vi "Exit.vi"(7 "Main VI":refnum<vi>, 8 "Error In":errorcluster, 9 "Messages":refnum<queue>, 10 "User Event In":refnum<user-event>, 11 "State In":T1) -> (0 "Error Out":errorcluster, 2 "User Event Out":refnum<user-event>, 3 "State Out":T1)   [LabVIEW 2018, in "Bookmark Manager.lvlib"]
uses:
  Bookmark Manager.lvlib
  Controls/State.ctl
  <vilib>/addons/analyzer/_analyzerctrls.llb/VIAnCtl Analysis App Info.ctl
  Controls/Bookmark.ctl
  Controls/VI Identifier.ctl
  Controls/Bookmarks Groups.ctl
  Controls/Message.ctl
  <vilib>/event_ctls.llb/usereventprio.ctl
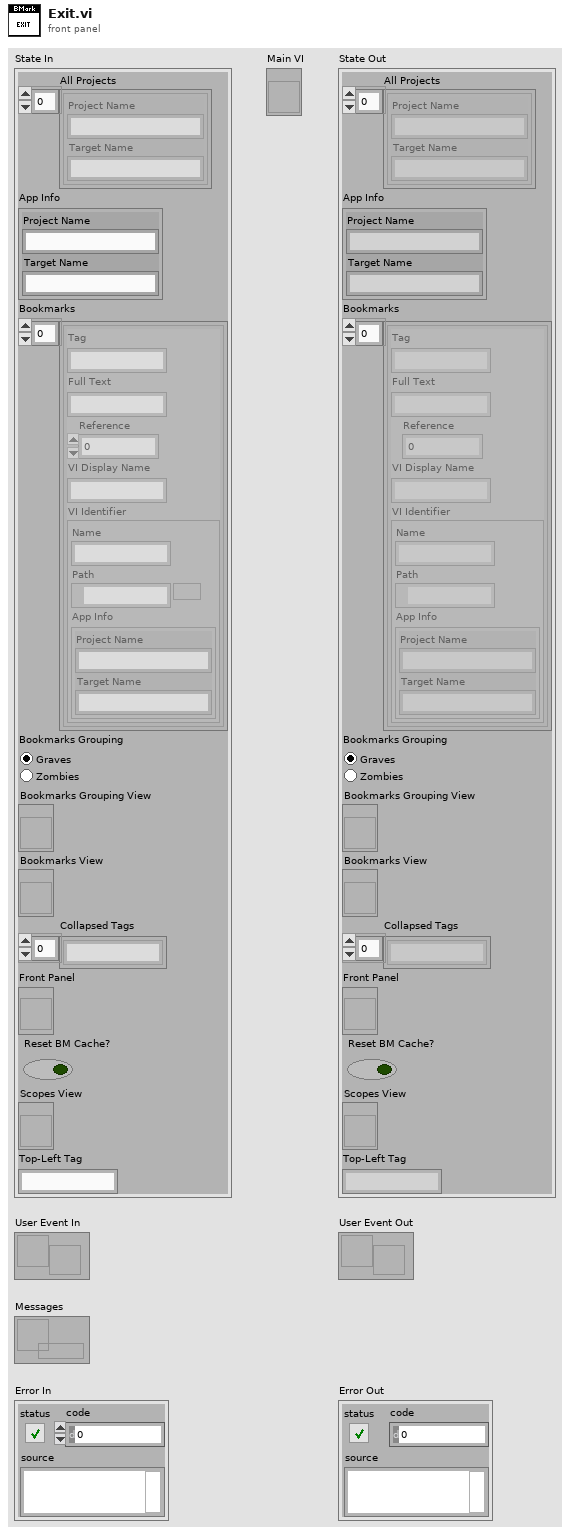
[diagram p1: front panel]
types:
  T1 = typedef "Bookmark Manager.lvlib/State.ctl" = cluster{"All Projects":T2[], "App Info":T2, "Bookmarks":T3[], "Bookmarks Grouping":T5, "Bookmarks Grouping View":refnum<vi>, "Bookmarks View":refnum<vi>, "Collapsed Tags":string[], "Front Panel":refnum<vi>, "Reset BM Cache?":bool, "Scopes View":refnum<vi>, "Top-Left Tag":string}
  T2 = typedef "VIAnCtl Analysis App Info.ctl" = cluster{"Project Name":string, "Target Name":string}
  T3 = typedef "Bookmark Manager.lvlib/Bookmark.ctl" = cluster{"Tag":string, "Full Text":string, "Reference":i32, "VI Display Name":string, "VI Identifier":T4}
  T4 = typedef "Bookmark Manager.lvlib/VI Identifier.ctl" = cluster{"Name":string, "Path":path, "App Info":T2}
  T5 = typedef "Bookmark Manager.lvlib/Bookmarks Groups.ctl" = enum32{"Graves", "Zombies"}
  T6 = typedef "usereventprio.ctl" = enum32{"high priority", "normal priority"}
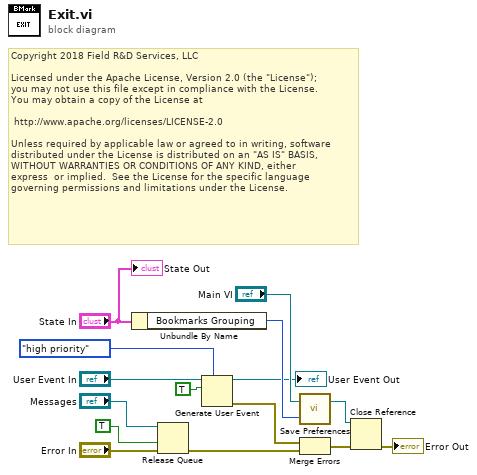
[diagram p0: block diagram]
diagram:
  # "Copyright 2018 Field R&D Services, LLC\n\nLicensed under the Apache License, Version 2.0 (the \"License\");\nyou may not use this file except in compliance with the License.\nYou may obtain a copy of the License at\n\n\thttp://www.apache.org/licenses/LICENSE-2.0\n\nUnless required by applicable law or agreed to in writing, software\ndistributed under the License is distributed on an \"AS IS\" BASIS,\nWITHOUT WARRANTIES OR CONDITIONS OF ANY KIND, either \nexpress  or implied.  See the License for the specific language \ngoverning permissions and limitations under the License."
  n1 = Unbundle By Name("State In") -> ("Bookmarks Grouping"=w11:T5)
  n2 = Release Queue(queue="Messages", force destroy? (F)=TRUE, error in (no error)="Error In") -> (error out=w9:errorcluster)  [unwired: 2 out]
  n3 = Generate User Event(priority (normal)=usereventprio."high priority", user event="User Event In", event data cluster=TRUE ("event data")) -> (user event out=→"User Event Out":refnum<user-event>, error out=w8:errorcluster)  [unwired: 1 in]
  n4 = call "Save Preferences.vi"("Bookmarks Groupings"=w11, "Graveyward Window In"="Main VI") -> ("Graveyard Window Out"=w13:refnum<vi>)  [unwired: 1 in]
  n5 = Merge Errors(w8, w9) -> (w14:errorcluster)
  n6 = Close Reference(reference=w13, error in (no error)=w14) -> (error out=→"Error Out":errorcluster)
  "State Out" <- "State In"
